vi "Test Set Active Rectangle.vi"(8 "error in (no error)":errorcluster) -> (0 "error out":errorcluster)   [LabVIEW 2019]
uses:
  <vilib>/addons/_JKI Toolkits/Caraya/classes/Assert/Assert.lvclass
  Setting Database/Setting Database.lvclass
  <vilib>/JKI/JKI SMO/SMO/SMO.lvclass
  <vilib>/addons/_JKI Toolkits/Caraya/classes/Test/Test.lvclass
  C:/Program Files (x86)/National Instruments/LabVIEW 2019/vi.lib/JKI/JKI SMO/SMO/SMO.lvclass
  Rectangle Settings/Rectangle Settings.lvclass
  <vilib>/addons/_JKI Toolkits/Caraya/classes/Assert/Assert Equal Value_Variant.vi
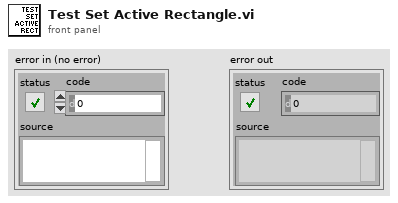
[diagram p1: front panel]
types:
  T1 = typedef "Setting Database.lvclass/PrivateEvents--Setting Database.Refresh.ctl" = cluster{"Paths":string[], "Rectangles":string[], "Funnels":string[], "Dots":string[]}
  T2 = typedef "Setting Database.lvclass/PublicEvents--Cluster.ctl" = cluster{"NewActivePath":refnum<user-event>, "PathsUpdated":refnum<user-event>, "RectanglesUpdated":refnum<user-event>, "NewActiveRectangle":refnum<user-event>, "NewActiveFunnel":refnum<user-event>, "FunnelsUpdated":refnum<user-event>, "NewActiveDot":refnum<user-event>, "DotsUpdated":refnum<user-event>}
  T3 = typedef "Setting Database.lvclass/PublicEvents--Setting Database.NewActiveRectangle.ctl" = refnum<class "Rectangle Settings.lvclass">
  T4 = typedef "Setting Database.lvclass/PublicEvents--Setting Database.RectanglesUpdated.ctl" = refnum<class "Rectangle Settings.lvclass">[]
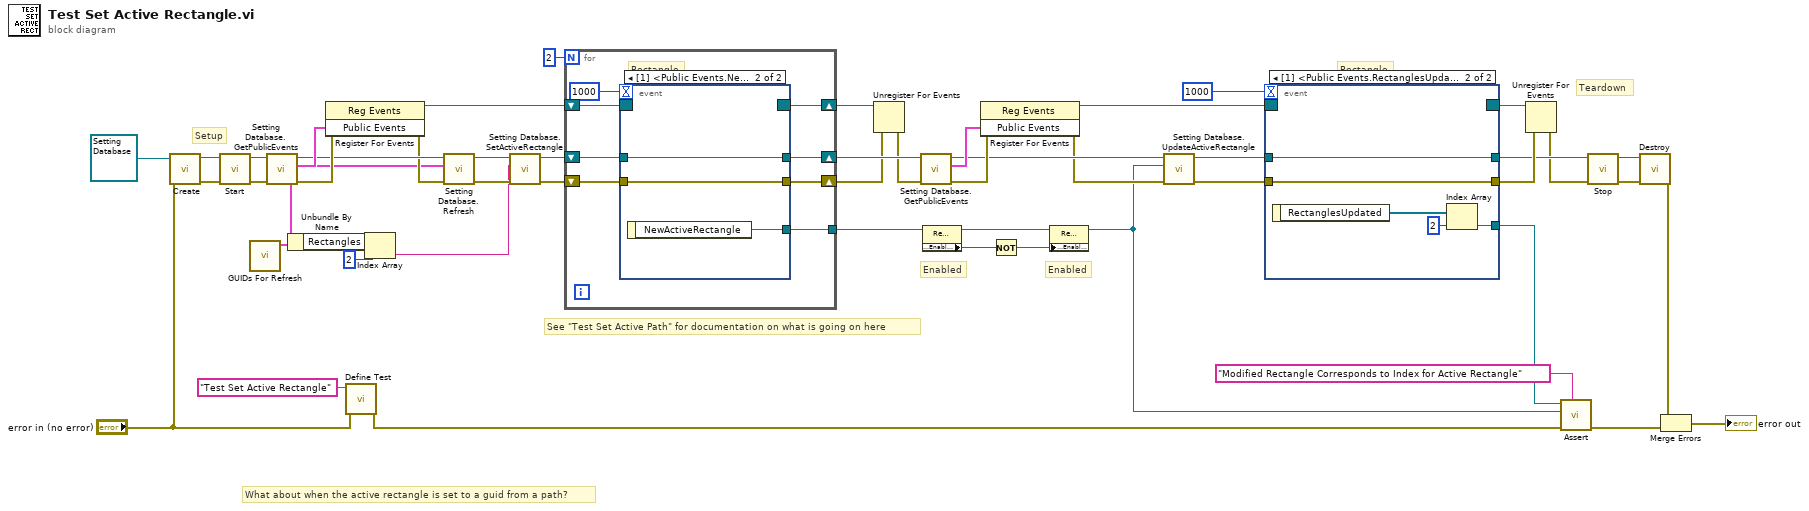
[diagram p0: block diagram]
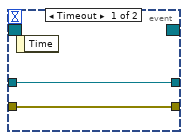
[diagram p2: hidden frame]
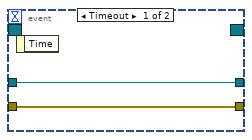
[diagram p3: hidden frame]
diagram:
  # "What about when the active rectangle is set to a guid from a path?"
  # "See \"Test Set Active Path\" for documentation on what is going on here"
  # "Enabled"
  # "Enabled"
  # "Rectangle"
  # "Teardown"
  # "Setup"
  n1 = call <vilib>:"Create.vi"("error in (no error)"="error in (no error)", "SMO"=refnum<class "Setting Database.lvclass"> refnum ("Setting Database.lvclass")) -> ("error out"=w48:errorcluster, "SMO out"=w42:refnum<class "Setting Database.lvclass">)  [unwired: 7 in, 1 out]
  n2 = call <vilib>:"Start.vi"("error in (no error)"=w48, "SMO"=w42) -> ("error out"=w47:errorcluster, "SMO out"=w41:refnum<class "Setting Database.lvclass">)  [unwired: 8 in]
  n3 = call "GUIDs For Refresh.vi"() -> ("Initialize"=w1:T1)  [unwired: 11 in]
  n4 = call "Setting Database.GetPublicEvents.vi"("error in (no error)"=w47, "Setting Database"=w41) -> ("error out"=w45:errorcluster, "Public Events"=w38:T2, "Setting Database out"=w36:refnum<class "Setting Database.lvclass">)  [unwired: 7 in]
  n5 = Unbundle By Name(w1) -> ("Rectangles"=w4:string[])
  n6 = register-events(error in=w45, w38) -> (reference out=w37:refnum<event-registration>, error out=w35:errorcluster)  [unwired: 1 in]
  n7 = call <vilib>:"Define Test.vi"("error in (no error)"="error in (no error)", "Label (VI Title)"="Test Set Active Rectangle") -> ("error out"=w11:errorcluster)  [unwired: 8 in, 1 out]
  n8 = Index Array(array=w4, index=2) -> (element=w2:string)
  n9 = call "Setting Database.Refresh.vi"("error in (no error)"=w35, "Initialize"=w1, "Setting Database"=w36) -> ("error out"=w6:errorcluster, "Setting Database out"=w8:refnum<class "Setting Database.lvclass">)  [unwired: 7 in]
  n10 = call "Setting Database.SetActiveRectangle.vi"("error in (no error)"=w6, "SetActiveRectangle"=w2, "Setting Database"=w8) -> ("error out"=w5:errorcluster, "Setting Database out"=w7:refnum<class "Setting Database.lvclass">)  [unwired: 7 in]
  n11 = for {
    N: 2 -> [_]
    tunnel: [w51] -> w23
    shift-right: [w58] -> w39
    shift-left: w37 -> [w56]
    shift-right: [w53] -> w34
    shift-left: w7 -> [w55]
    shift-right: [w52] -> w33
    shift-left: w5 -> [w54]
    # "Rectangle"
    n12 = event shown="[1] <Public Events.NewActiveRectangle>: User Event" {
      selector: w56 -> [_ _]
      dyn-events: [_ _] -> w58
      timeout: 1000 -> [_ _]
      tunnel: [w60 w63] -> w52
      tunnel: w54 -> [w60 w63]
      tunnel: w55 -> [w59 w62]
      tunnel: [w59 w62] -> w53
      tunnel: [_ w61] -> w51
      event Timeout {
        n13 = event-data() -> ()  [unwired: 1 in, 1 out]
      }
      event User Event {
        n14 = event-data() -> ("NewActiveRectangle"=w61:T3)  [unwired: 1 in]
      }
    }
  }
  n15 = Unregister For Events(event registration refnum=w39, error in=w33) -> (error out=w32:errorcluster)
  n16 = call "Setting Database.GetPublicEvents.vi"("error in (no error)"=w32, "Setting Database"=w34) -> ("error out"=w30:errorcluster, "Public Events"=w31:T2, "Setting Database out"=w17:refnum<class "Setting Database.lvclass">)  [unwired: 7 in]
  n17 = property class="Rectangle Settings.lvclass"(reference=w23) -> (reference out=w22:T3, "Accessors:Enabled"=w21:bool)  [unwired: 1 in, 1 out]
  n18 = register-events(error in=w30, w31) -> (reference out=w26:refnum<event-registration>, error out=w15:errorcluster)  [unwired: 1 in]
  n19 = Not(x=w21) -> (.not. x?=w20:bool)
  n20 = property class="Rectangle Settings.lvclass"(reference=w22, "Accessors:Enabled"=w20) -> (reference out=w13:T3)  [unwired: 1 in, 1 out]
  n21 = call "Setting Database.UpdateActiveRectangle.vi"("error in (no error)"=w15, "UpdateActiveRectangle"=w13, "Setting Database"=w17) -> ("error out"=w14:errorcluster, "Setting Database"=w16:refnum<class "Setting Database.lvclass">)  [unwired: 7 in]
  n22 = event shown="[1] <Public Events.RectanglesUpdated>: User Event" {
    selector: w26 -> [_ _]
    dyn-events: [_ _] -> w27
    timeout: 1000 -> [_ _]
    tunnel: [w65 w70] -> w29
    tunnel: w14 -> [w65 w70]
    tunnel: w16 -> [w64 w69]
    tunnel: [w64 w69] -> w25
    tunnel: [_ w67] -> w19
    event Timeout {
      n23 = event-data() -> ()  [unwired: 1 in, 1 out]
    }
    event User Event {
      n24 = event-data() -> ("RectanglesUpdated"=w68:T4)  [unwired: 1 in]
      n25 = Index Array(array=w68, index=2) -> (element=w67:refnum<class "Rectangle Settings.lvclass">)
    }
  }
  n26 = Unregister For Events(event registration refnum=w27, error in=w29) -> (error out=w24:errorcluster)
  n27 = call-poly <vilib>:"Assert.vi"("Label"="Modified Rectangle Corresponds to Index for Active Rectangle", "error in (no error)"=w11, "Actual"=w13, "Expected"=w19) -> ("error out"=w50:errorcluster)  [unwired: 6 in, 1 out]
  n28 = call <vilib>:"Stop.vi"("error in (no error)"=w24, "SMO"=w25) -> ("error out"=w46:errorcluster, "SMO out"=w40:refnum<class "Setting Database.lvclass">)  [unwired: 8 in]
  n29 = call <vilib>:"Destroy.vi"("error in (no error)"=w46, "SMO"=w40) -> ("error out"=w44:errorcluster)  [unwired: 9 in]
  n30 = Merge Errors(w44, w50) -> (→"error out":errorcluster)
